vi "SVPO Convert to Even Angle Signal (N Ch DBL Array).vi"(0 "scaled signals [EU]":dbl[][](array[numeric]), 2 "reset? (F)":bool, 5 "sampling rate [Hz]":dbl=1.0, 7 "speed position info":T1, 12 "max order":dbl=16.0) -> (4 "even-angle signals":cluster{"r0":dbl, "dr":dbl, "Y":dbl[]}[](array[cluster]) {"r0" format="%.2p"; "dr" format="%.2p"; "Y" format="%.2f"}, 8 "even-angle position info":T1)   [LabVIEW 2017, in "SoundVib_OrderTracking.lvlib"]
doc: "Converts an even-time-spaced scaled signal to an even-angle-spaced signal by resampling the acquired signal. The output signal is synchronous to the rotational speed with a constant number of samples per revolution. Use this VI on embedded targets that have limited computational resources. Wire data to the <B>scaled signal [EU]</B> input to determine the polymorphic instance to use or manually select the instance."
uses:
  <vilib>/addons/Sound and Vibration/Order Analysis/Resample Order Tracking/SoundVib_OrderTracking.lvlib
  <vilib>/addons/Sound and Vibration/Order Analysis/Misc/OAT Position Info.ctl
  <vilib>/addons/Sound and Vibration/Order Analysis/Adv Resampling/oa_CIC Interpolation Filter with IC.vi
  <vilib>/addons/Sound and Vibration/Order Analysis/Adv Resampling/sv_Resample (Const to Variable, DBL Array) with IC.vi
  <vilib>/addons/Sound and Vibration/Order Analysis/Adv Resampling/sv_Resample Filter Prototype Design.vi
  <vilib>/addons/Sound and Vibration/Order Analysis/Adv Resampling/oa_Adjust Resample State Info.vi
  <vilib>/addons/Sound and Vibration/Order Analysis/Adv Resampling/OAT LP Kaiser Window Design.vi
  <vilib>/addons/Sound and Vibration/Order Analysis/Resample Order Tracking/SubVIs/oa_CIC Filter Length.vi
  <vilib>/addons/Sound and Vibration/Order Analysis/Adv Resampling/sv_Get Actual Max Order.vi
  <vilib>/addons/Sound and Vibration/Order Analysis/Resample Order Tracking/SoundVib_Resampling.lvlib
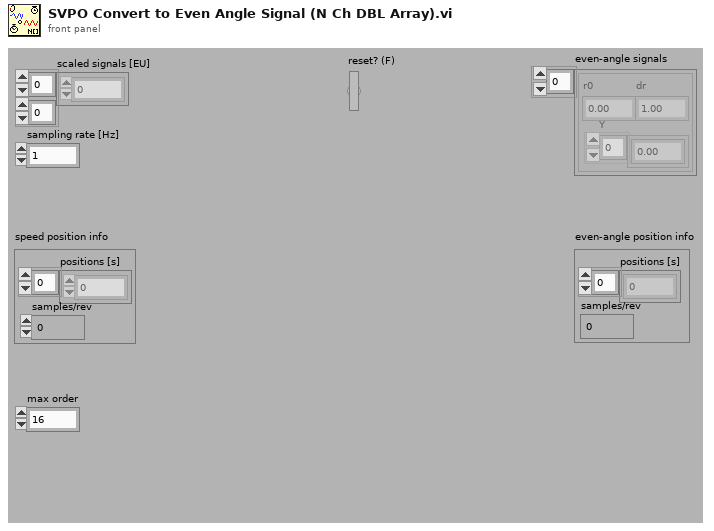
[diagram p1: front panel]
types:
  T1 = typedef "OAT Position Info.ctl" = cluster{"positions [s]":dbl[], "samples/rev":dbl}
  T2 = typedef "svc_Convert to Even Angle State.ctl" = cluster{"filter prototype":T3, "interpolation filter state":cluster{"corrected lengths":i32[], "initH":cluster{"t":dbl[]}[]}, "resample state":cluster{"signal length":u64, "time":dbl[], "reset state":bool, "state":cluster{"init condition":dbl[], "start index":i32, "channel count":i32, "condition len":i32, "position":dbl, "time interval":dbl, "max cond len":i32}, "offset":dbl}}
  T3 = typedef "OAT Resample Filter Prototype.ctl" = cluster{"left wing":dbl[], "increment":dbl[], "max dec":i32, "timing jitter":enum32{"Interpolation", "Rounding"}, "band limiting?":bool}
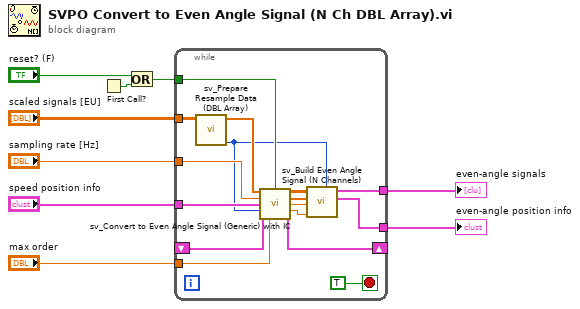
[diagram p0: block diagram]
diagram:
  n1 = First Call?() -> (First Call?: T/F=w6:bool)
  n2 = Or(x="reset? (F)", y=w6) -> (x .or. y?=w4:bool)
  n3 = while {
    tunnel: [w25] -> w9
    tunnel: [w24] -> w8
    tunnel: "scaled signals [EU]" -> [w23]
    tunnel: w4 -> [w21]
    tunnel: "sampling rate [Hz]" -> [w20]
    tunnel: "speed position info" -> [w19]
    tunnel: "max order" -> [w18]
    shift-right: [w13] -> _
    shift-left: _ -> [w12]
    stop <- TRUE stop-if-true
    n4 = call <vilib>:"sv_Prepare Resample Data (DBL Array).vi"("Array"=w23) -> ("channel count"=w10:i32, "Y"=w22:dbl[])  [unwired: 8 in, 1 out]
    n5 = call <vilib>:"sv_Convert to Even Angle Signal (Generic) with IC.vi"("scaled signal [EU]"=w22, "reset? (F)"=w21, "sampling rate [Hz]"=w20, "speed position info"=w19, "channel count"=w10, "initial conditions"=w12, "max order"=w18) -> ("generic even-angle signal"=w17:dbl[][], "generic position info"=w16:dbl[], "offset"=w15:dbl, "pulse/revolution"=w14:dbl, "final conditions"=w13:T2)  [unwired: 4 in]
    n6 = call <vilib>:"sv_Build Even Angle Signal (N Channels).vi"("# of ch"=w10, "samples/rev"=w14, "offset"=w15, "time stamps"=w16, "Data"=w17) -> ("even-angle position info"=w24:T1, "even-angle signals"=w25:cluster{"r0":dbl, "dr":dbl, "Y":dbl[]}[])  [unwired: 5 in]
  }
  "even-angle position info" <- w8
  "even-angle signals" <- w9
